vi "4Pi 4Pi Modes - Compute Voltage.vi"() -> ()   [LabVIEW 2016]
panel:
  out "Voltage":dbl[](array[numeric])
  in  "Norm Voltage (-1 to 1)":dbl[](array[numeric])
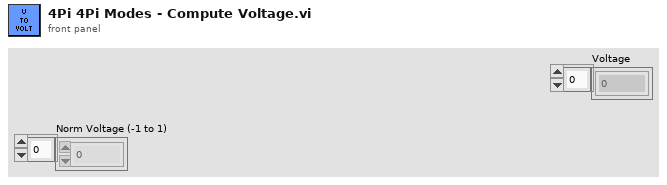
[diagram p1: front panel]
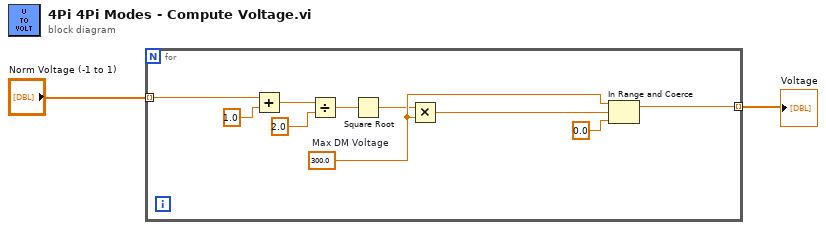
[diagram p0: block diagram]
diagram:
  n1 = for {
    tunnel: "Norm Voltage (-1 to 1)" -> [w5] mode=indexing
    tunnel: [w4] -> w1 mode=indexing
    w12 = 300.0  # Max DM Voltage
    n2 = Add(x=w5, y=1.0) -> (x+y=w7:dbl)
    n3 = Divide(x=w7, y=2.0) -> (x/y=w9:dbl)
    n4 = Square Root(x=w9) -> (sqrt(x)=w10:dbl)
    n5 = Multiply(x=w10, y=w12) -> (x*y=w3:dbl)
    n6 = In Range and Coerce(upper limit=w12, x=w3, lower limit=0.0) -> (coerced(x)=w4:dbl)  [unwired: 1 out]
  }
  "Voltage" <- w1
